vi "PusherGetPosition.vi"() -> ()   [LabVIEW 2014, in "PusherLib.lvlib"]
uses:
  PusherLib.lvlib
panel:
  out "PusherPositionActual":dbl
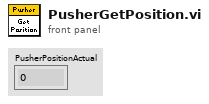
[diagram p1: front panel]
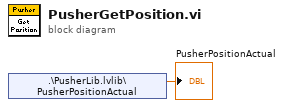
[diagram p0: block diagram]
diagram:
  n1 = shared-variable ".\\PusherLib.lvlib\\PusherPositionActual"() -> (→"PusherPositionActual":dbl)  [unwired: 1 in, 1 out]
